vi "RT Driver VI.vi"(7 "Operation":T1, 11 "Device Reference in":T2 format="%.0x") -> (0 "Error Code":i32)   [LabVIEW 2015, in "SLSC-12201 DIO Engine.lvlib"]
uses:
  SLSC-12201 DIO Engine.lvlib
  <vilib>/NI Veristand/Custom Device API/Custom Device Item Ref.ctl
  <vilib>/NI Veristand/Custom Device API/Hardware Interface Driver VI Operation.ctl
  Shared/Compiled.Settings
  Shared/SLSC Dynamic Channel.ctl
  Shared/SLSC Dynamic Channel Type.ctl
  Types/RTStateVariables.ctl
  <vilib>/NI/NIVS Inline Async API/_VS Inline Async API/VS Inline Async API/VS Inline Async API.lvclass
  <vilib>/NI/NIVS Inline Async API/_VS Inline Async API/VS Inline Async API/VS Inline Async API.lvclass/VS Inline Async API.ctl
  <vilib>/NI/NIVS Inline Async API/_Data Access Engine/Data Access Engine/Data Access Engine.lvclass/Data Access Engine.ctl
  <vilib>/NI/NIVS Inline Async API/_Data Access Engine/Access Type Classes/Write/Write.lvclass/Write.ctl
  <vilib>/NI/NIVS Inline Async API/_Data Access Engine/Access Type Classes/ReadWrite/ReadWrite.lvclass/ReadWrite.ctl
  <vilib>/NI/NIVS Inline Async API/_Data Access Engine/Access Type Classes/Read/Read.lvclass/Read.ctl
  <vilib>/NI/NIVS Inline Async API/_Data Access Engine/Data Access Engine/Methods/Data.Engine.Read Data from HW.vi
  <vilib>/NI/NIVS Inline Async API/_VS Inline Async API/Error Handling Process/SubVIs/Error.GetError.vi
  <vilib>/NI/NIVS Inline Async API/_Data Access Engine/Data Access Engine/Methods/Data.Engine.Write Data to HW.vi
  <vilib>/NI/NIVS Inline Async API/_Data Access Engine/Access Type Classes/ReadWrite/ReadWrite.EngineData.vi
  <vilib>/NI/NIVS Inline Async API/_Data Access Engine/Access Type Classes/Write/Write.EngineData.vi
  <vilib>/NI/NIVS Inline Async API/_Data Access Engine/Access Type Classes/Read/Read.EngineData.vi
  <vilib>/NI Veristand/Custom Device API/NI VeriStand - Get Channel Value by Data Reference.vi
  <vilib>/NI Veristand/Custom Device API/NI VeriStand - Set Channel Value by Data Reference.vi
  <vilib>/NI Veristand/Custom Device API/NI VeriStand - Get Channel Values by Block Data Reference.vi
  Shared/Constants.vi
  <vilib>/NI Veristand/Custom Device API/Get Item Property (Variant).vi
  <vilib>/NI Veristand/Custom Device API/Global Data Refs.vi
  <vilib>/NI Veristand/Custom Device API/Custom Device API.lvlib
  Shared/SLSC-12201 DIO Shared.lvlib
  <vilib>/NI Veristand/Custom Device Tools/Custom Device Utility Library/Custom Device Utility Library.lvlib
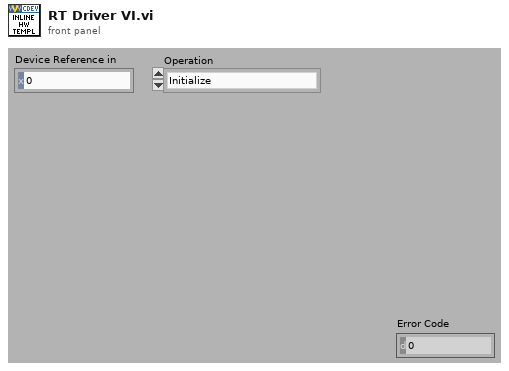
[diagram p1: front panel]
types:
  T1 = typedef "Custom Device API.lvlib/Hardware Interface Driver VI Operation.ctl" = enum16{"Initialize", "Start", "Read Data from HW", "Write Data to HW", "Close"}
  T2 = typedef "Custom Device API.lvlib/Custom Device Item Ref.ctl" = u64
  T3 = typedef "SLSC-12201 DIO Engine.lvlib/RTStateVariables.ctl" = cluster{"Async":refnum<class "VS Inline Async API.lvclass">, "Settings":T4}
  T4 = typedef "SLSC-12201 DIO Shared.lvlib/Compiled.Settings" = cluster{"Name":string, "SLSC IP -Module Name":string, "Slot #":i32, "Configuration Data":cluster{"Properties":cluster{"Boolean Properties":cluster{"property":refnum<k21>, "Value":bool, "SLSC Item":refnum<k21>}[], "Double Properties":cluster{"property":refnum<k21>, "Double Write":dbl, "SLSC Item":refnum<k21>}[], "I32 Properties":cluster{"property":refnum<k21>, "Int32 Write":i32, "SLSC Item":refnum<k21>}[], "I64 Properties":cluster{"property":refnum<k21>, "Int64 Write":i64, "SLSC Item":refnum<k21>}[], "String Properties":cluster{"property":refnum<k21>, "String Write":string, "SLSC Item":refnum<k21>}[], "U32 Properties":cluster{"property":refnum<k21>, "UInt32 Write":u32, "SLSC Item":refnum<k21>}[], "U64 Properties":cluster{"property":refnum<k21>, "UInt64 Write":u64, "SLSC Item":refnum<k21>}[]}}, "SLSC Set Properties":T5[], "SLSC Get Properties":T5[], "SLSC Commands":T5[], "Username":string, "Password":string, "Support Modules":cluster{"Dev.ProductNumber":u32, "Dev.VendorNumber":u32}[]}
  T5 = typedef "SLSC-12201 DIO Shared.lvlib/SLSC Dynamic Channel.ctl" = cluster{"SLSC Item":string, "property":string, "Data Type":T6, "Value":variant}
  T6 = typedef "SLSC-12201 DIO Shared.lvlib/SLSC Dynamic Channel Type.ctl" = enum16{"Bool", "Double", "I32", "I64", "String", "U32", "U64", "EnumI32"}
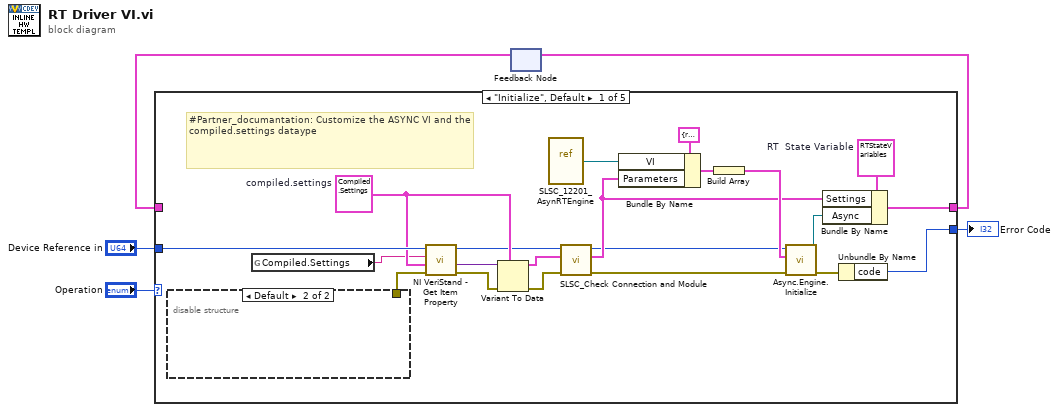
[diagram p0: block diagram]
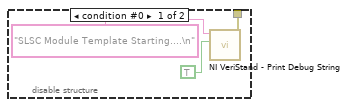
[diagram p2: hidden frame]
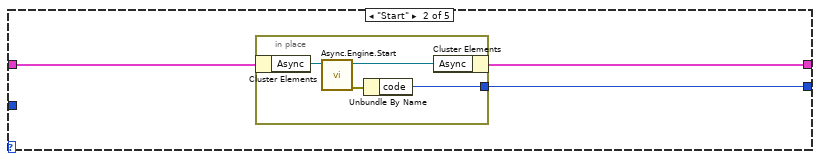
[diagram p3: hidden frame]
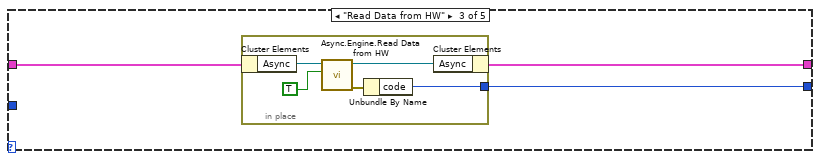
[diagram p4: hidden frame]
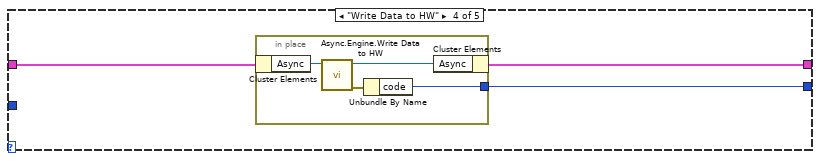
[diagram p5: hidden frame]
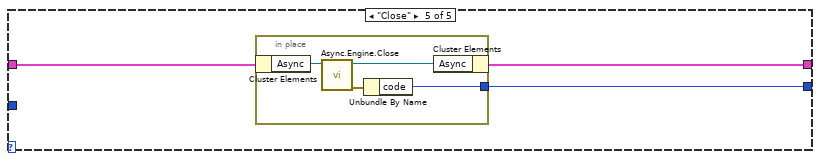
[diagram p6: hidden frame]
diagram:
  n1 = feedback #1() -> (w3:T3)  [unwired: 1 out]
  n2 = case shown="\"Initialize\", Default" "Operation" {
    tunnel: [w24 w31 w37 w45 w53] -> w4
    tunnel: w3 -> [_ w32 w39 w46 w54]
    tunnel: "Device Reference in" -> [w21 _ _ _ _]
    tunnel: [w26 w30 w38 w47 w52] -> w1
    frame "Initialize", Default {
      w16 = T3 {"Async"=refnum, "Settings"={"Name"="", "SLSC IP -Module Name"="", "Slot #"=0, "Configuration Data"={"Properties"={"Boolean Properties"=[], "Double Properties"=[], "I32 Properties"=[], "I64 Properties"=[], "String Properties"=[], "U32 Properties"=[], "U64 Properties"=[]}}, "SLSC Set Properties"=[], "SLSC Get Properties"=[], "SLSC Commands"=[], "Username"="", "Password"="", "Support Modules"=[]}}  # RT  State Variable
      w17 = T4 {"Name"="", "SLSC IP -Module Name"="", "Slot #"=0, "Configuration Data"={"Properties"={"Boolean Properties"=[], "Double Properties"=[], "I32 Properties"=[], "I64 Properties"=[], "String Properties"=[], "U32 Properties"=[], "U64 Properties"=[]}}, "SLSC Set Properties"=[], "SLSC Get Properties"=[], "SLSC Commands"=[], "Username"="", "Password"="", "Support Modules"=[]}  # compiled.settings
      # "#Partner_documantation: Customize the ASYNC VI and the compiled.settings dataype"
      n3 = disable-structure shown="Default" {
        disable-tunnel: [w29 _] -> w14
        frame condition #0 {
          n4 = call <vilib>:"NI VeriStand - Print Debug String.vi"("Add to log file? (T)"=TRUE, "Message"="SLSC Module Template Starting....\n") -> ("error out"=w29:errorcluster)  [unwired: 9 in]
        }
        frame condition #1 (active) {
        }
      }
      n5 = global read "Constants.vi" "Compiled.Settings"() -> (w13:string)
      n6 = call-poly <vilib>:"NI VeriStand - Get Item Property.vi"("error in (no error)"=w14, "Default Value"=w17, "Property Name"=w13, "Item Ref in"=w21) -> ("error out"=w20:errorcluster, "Value"=w19:variant, "Item Ref out"=w7:T2)  [unwired: 4 in, 1 out]
      n7 = Variant To Data(error in=w20, type=w17, Variant=w19) -> (data=w9:T4, error out=w11:errorcluster)
      n8 = vi-ref "SLSC_12201_AsynRTEngine.vi"() -> (w12:refnum<vi>)
      n9 = call "SLSC_Check Connection and Module.vi"("error in (no error)"=w11, "compiled.settings"=w9, "Item Ref in"=w7) -> ("error out"=w10:errorcluster, "compiled.settings out"=w8:T4, "Item Ref out"=w6:T2)  [unwired: 5 in, 1 out]
      n10 = Bundle By Name(cluster=cluster{"VI":refnum<vi>, "Parameters":variant} {"VI"=refnum, "Parameters"=variant} ("Process"), "VI"=w12, "Parameters"=w8) -> (w22:cluster{"VI":refnum<vi>, "Parameters":variant})
      n11 = Build Array(w22) -> (w15:cluster{"VI":refnum<vi>, "Parameters":variant}[])
      n12 = call <vilib>:"Async.Engine.Initialize.vi"("error in (no error)"=w10, "Processes"=w15, "Custom Device Ref"=w6) -> ("error out"=w18:errorcluster, "Async"=w25:refnum<class "VS Inline Async API.lvclass">)  [unwired: 7 in]
      n13 = Bundle By Name(cluster=w16, "Settings"=w8, "Async"=w25) -> (w24:T3)
      n14 = Unbundle By Name(w18) -> ("code"=w26:i32)
    }
    frame "Start" {
      n15 = in-place {
        in-place-border: [w33] -> w30
        n16 = in-place-cluster #2(w32) -> ("Async"=w36:refnum<class "VS Inline Async API.lvclass">)
        n17 = call <vilib>:"Async.Engine.Start.vi"("VS Inline Async API in"=w36) -> ("error out"=w34:errorcluster, "VS Inline Async API out"=w35:refnum<class "VS Inline Async API.lvclass">)  [unwired: 9 in]
        n18 = Unbundle By Name(w34) -> ("code"=w33:i32)
        n19 = in-place-cluster #2("Async"=w35) -> (w31:T3)
      }
    }
    frame "Read Data from HW" {
      n20 = in-place {
        in-place-border: [w42] -> w38
        n21 = in-place-cluster #3(w39) -> ("Async"=w44:refnum<class "VS Inline Async API.lvclass">)
        n22 = call <vilib>:"Async.Engine.Read Data from HW.vi"("Report Error to Inline?"=TRUE, "Async in"=w44) -> ("error out"=w41:errorcluster, "Async out"=w43:refnum<class "VS Inline Async API.lvclass">)  [unwired: 8 in]
        n23 = Unbundle By Name(w41) -> ("code"=w42:i32)
        n24 = in-place-cluster #3("Async"=w43) -> (w37:T3)
      }
    }
    frame "Write Data to HW" {
      n25 = in-place {
        in-place-border: [w51] -> w47
        n26 = in-place-cluster #4(w46) -> ("Async"=w49:refnum<class "VS Inline Async API.lvclass">)
        n27 = call <vilib>:"Async.Engine.Write Data to HW.vi"("VS Inline Async API in"=w49) -> ("error out"=w50:errorcluster, "VS Inline Async API out"=w48:refnum<class "VS Inline Async API.lvclass">)  [unwired: 9 in]
        n28 = Unbundle By Name(w50) -> ("code"=w51:i32)
        n29 = in-place-cluster #4("Async"=w48) -> (w45:T3)
      }
    }
    frame "Close" {
      n30 = in-place {
        in-place-border: [w56] -> w52
        n31 = in-place-cluster #5(w54) -> ("Async"=w58:refnum<class "VS Inline Async API.lvclass">)
        n32 = call <vilib>:"Async.Engine.Close.vi"("Async in"=w58) -> ("error out"=w55:errorcluster, "Async out"=w57:refnum<class "VS Inline Async API.lvclass">)  [unwired: 9 in]
        n33 = Unbundle By Name(w55) -> ("code"=w56:i32)
        n34 = in-place-cluster #5("Async"=w57) -> (w53:T3)
      }
    }
  }
  "Error Code" <- w1
  n35 = feedback-in #1(w4) -> ()
